vi "Main Voice.vi"() -> ()   [LabVIEW 2018]
uses:
  <vilib>/LabVIEW Hacker/LINX/Private/Type Defs/User Platform.ctl
  <vilib>/LabVIEW Hacker/LINX/Private/Type Defs/Interface.ctl
  <vilib>/LabVIEW Hacker/LINX/Public/Peripherals/Digital/Digital Write 1 Chan.vi
  <vilib>/LabVIEW Hacker/LINX/Public/Peripherals/Digital/Digital Write N Chans.vi
  <vilib>/LabVIEW Hacker/LINX/Private/Local IO/LinxDigitalWrite.vi
  <vilib>/LabVIEW Hacker/LINX/Public/Utilities/Check Channel.vi
  <vilib>/LabVIEW Hacker/LINX/Private/Utilties/Generate Error.vi
  <vilib>/LabVIEW Hacker/LINX/LMH-LINX.lvlib
panel:
  out "Command":string[](array[string])
  in  "Error In":errorcluster
  out "Error Out":errorcluster
  in  "Exit":bool
  out "Voice Command":string
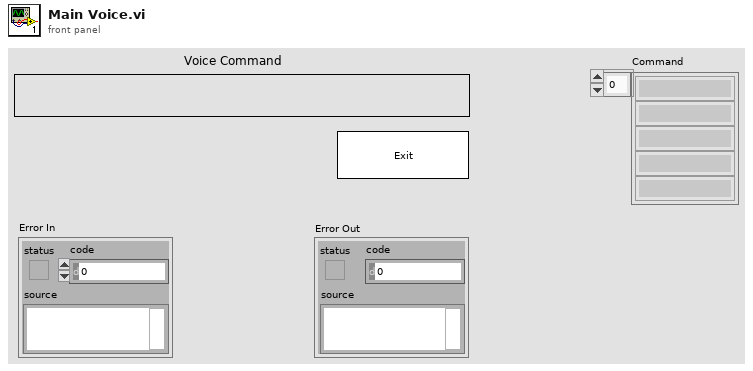
[diagram p1: front panel]
types:
  T1 = typedef "LMH-LINX.lvlib/Interface.ctl" = enum16{"Serial", "TCP"}
  T2 = typedef "LMH-LINX.lvlib/User Platform.ctl" = enum16{"Default", "Remote", "Local"}
  T3 = typedef "LMH-LINX.lvlib/LINX Ref.ctl" = cluster{"IO":T4, "Interface":T1, "LINX Device Config":T5}
  T4 = typedef "LMH-LINX.lvlib/Platform.ctl" = enum16{"Remote", "Local"}
  T5 = typedef "LMH-LINX.lvlib/Device.lvlib/LINX Device Config.ctl" = cluster{"Interface":T1, "COM Port":refnum<visa-resource-name>, "TCP Configuration":T6, "Device Family":u8, "Device ID":u8, "Device Name":string, "TCP Ref":refnum<k5>, "Channels":T7}
  T6 = typedef "LMH-LINX.lvlib/Device.lvlib/TCP Config.ctl" = cluster{"IP Address":string, "Port":u16}
  T7 = typedef "LMH-LINX.lvlib/Channels.ctl" = cluster{"DI":u8[], "DO":u8[], "AI":u8[], "AO":u8[], "PWM":u8[], "QE":u8[], "UART":u8[], "I2C 2":u8[], "SPI":u8[], "CAN":u8[], "Servo":u8[], "AI Ref (V)":dbl, "AI Resolution (Bits)":u8, "AO Ref (V)":dbl, "AO Resolution (Bits)":u8}
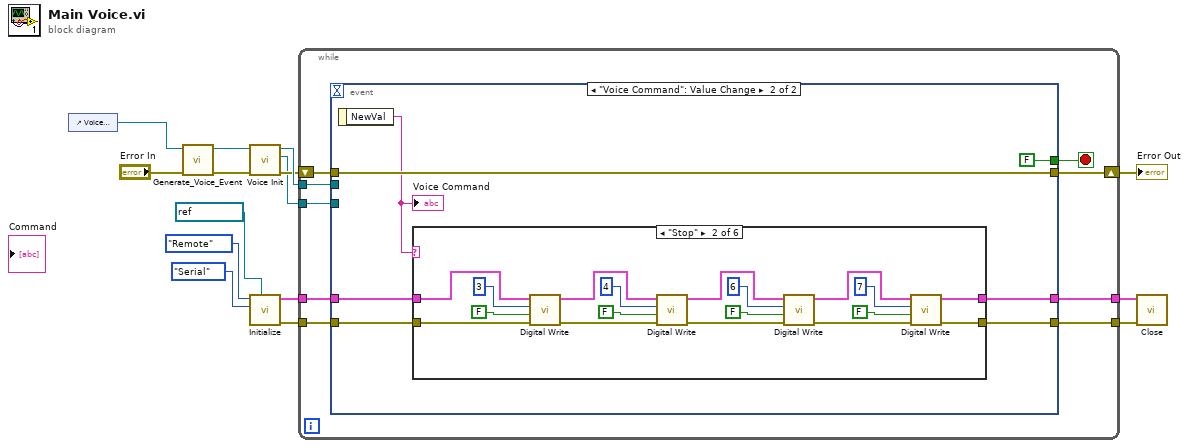
[diagram p0: block diagram]
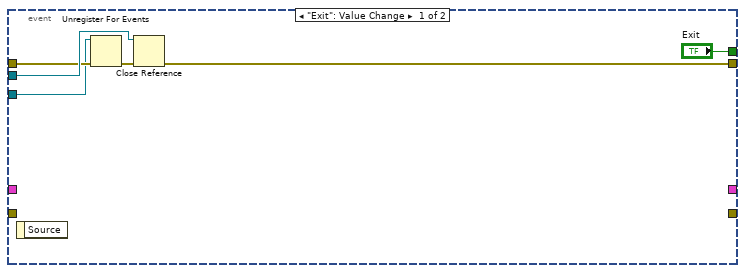
[diagram p2: hidden frame]
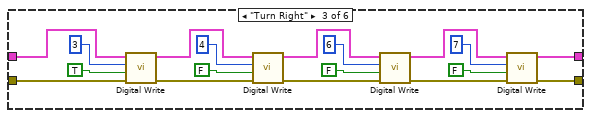
[diagram p4: hidden frame]
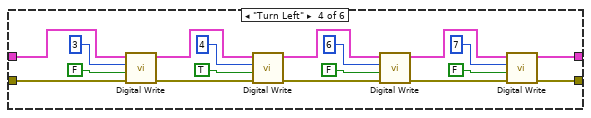
[diagram p5: hidden frame]
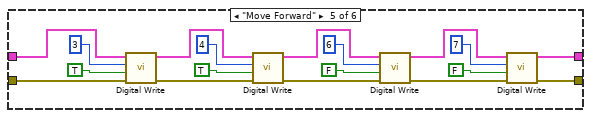
[diagram p6: hidden frame]
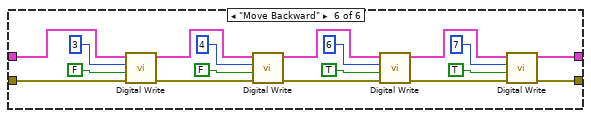
[diagram p7: hidden frame]
diagram:
  n1 = control-ref of="Voice Command"() -> (w14:refnum<vi>)
  n2 = call "Generate_Voice_Event.vi"("Error In"="Error In", "String in"=w14) -> ("Error Out"=w13:errorcluster, "String out"=w15:refnum<vi>)  [unwired: 8 in]
  n3 = call "Voice Init.vi"("Error In"=w13, "Text"=w15) -> ("Error Out"=w11:errorcluster, "Event Callback"=w8:refnum<k27>, "Reference"=w12:refnum<k24>)  [unwired: 7 in]
  n4 = call <vilib>:"Initialize.vi"("Serial Port"=refnum<visa-resource-name> "COM19", "Interface"=Interface."Serial", "IO"=User_Platform."Remote" ("Platform")) -> ("Error Out"=w6:errorcluster, "LINX Resource"=w7:T3)  [unwired: 6 in, 1 out]
  n5 = while {
    tunnel: w12 -> [w23]
    shift-right: [w21] -> w10
    shift-left: w11 -> [w22]
    tunnel: w8 -> [w20]
    tunnel: w7 -> [w19]
    tunnel: w6 -> [w18]
    tunnel: [w17] -> w5
    tunnel: [w16] -> w4
    stop <- w24 stop-if-true
    n6 = event shown="[1] \"Voice Command\": Value Change" {
      selector: _ -> [_ _]
      dyn-events: _ -> [_ _]
      timeout: _ -> [_ _]
      tunnel: ["Exit" FALSE ("Exit")] -> w24
      tunnel: w23 -> [w29 _]
      tunnel: w22 -> [w27 w37]
      tunnel: [w26 w37] -> w21
      tunnel: w20 -> [w25 _]
      tunnel: w19 -> [_ w34]
      tunnel: w18 -> [_ w33]
      tunnel: [_ w32] -> w17
      tunnel: [_ w31] -> w16
      event "Exit": Value Change {
        n7 = event-data() -> ()  [unwired: 1 in, 1 out]
        n8 = Unregister For Events(event registration refnum=w25, error in=w27) -> (error out=w28:errorcluster)
        n9 = Close Reference(reference=w29, error in (no error)=w28) -> (error out=w26:errorcluster)
      }
      event "Voice Command": Value Change {
        n10 = event-data() -> ("NewVal"=w35:string)  [unwired: 1 in]
        "Voice Command" <- w35
        n11 = case shown="\"Stop\"" w35 {
          tunnel: w34 -> [w39 w46 w64 w82 w100 w118]
          tunnel: w33 -> [w38 w45 w63 w81 w99 w117]
          tunnel: [w39 w41 w62 w77 w95 w113] -> w32
          tunnel: [w38 w40 w61 w76 w94 w112] -> w31
          frame Default {
          }
          frame "Stop" {
            n12 = call-poly <vilib>:"Digital Write.vi"("Error In"=w45, "Output Value"=FALSE, "DO Channel"=u8 3, "LINX Resource"=w46) -> ("Error Out"=w44:errorcluster, "LINX Resource"=w47:T3)  [unwired: 6 in]
            n13 = call-poly <vilib>:"Digital Write.vi"("Error In"=w44, "Output Value"=FALSE, "DO Channel"=u8 4, "LINX Resource"=w47) -> ("Error Out"=w43:errorcluster, "LINX Resource"=w48:T3)  [unwired: 6 in]
            n14 = call-poly <vilib>:"Digital Write.vi"("Error In"=w43, "Output Value"=FALSE, "DO Channel"=u8 6, "LINX Resource"=w48) -> ("Error Out"=w42:errorcluster, "LINX Resource"=w49:T3)  [unwired: 6 in]
            n15 = call-poly <vilib>:"Digital Write.vi"("Error In"=w42, "Output Value"=FALSE, "DO Channel"=u8 7, "LINX Resource"=w49) -> ("Error Out"=w40:errorcluster, "LINX Resource"=w41:T3)  [unwired: 6 in]
          }
          frame "Turn Right" {
            n16 = call-poly <vilib>:"Digital Write.vi"("Error In"=w63, "Output Value"=TRUE, "DO Channel"=u8 3, "LINX Resource"=w64) -> ("Error Out"=w60:errorcluster, "LINX Resource"=w75:T3)  [unwired: 6 in]
            n17 = call-poly <vilib>:"Digital Write.vi"("Error In"=w60, "Output Value"=FALSE, "DO Channel"=u8 4, "LINX Resource"=w75) -> ("Error Out"=w59:errorcluster, "LINX Resource"=w74:T3)  [unwired: 6 in]
            n18 = call-poly <vilib>:"Digital Write.vi"("Error In"=w59, "Output Value"=FALSE, "DO Channel"=u8 6, "LINX Resource"=w74) -> ("Error Out"=w58:errorcluster, "LINX Resource"=w73:T3)  [unwired: 6 in]
            n19 = call-poly <vilib>:"Digital Write.vi"("Error In"=w58, "Output Value"=FALSE, "DO Channel"=u8 7, "LINX Resource"=w73) -> ("Error Out"=w61:errorcluster, "LINX Resource"=w62:T3)  [unwired: 6 in]
          }
          frame "Turn Left" {
            n20 = call-poly <vilib>:"Digital Write.vi"("Error In"=w81, "Output Value"=FALSE, "DO Channel"=u8 3, "LINX Resource"=w82) -> ("Error Out"=w80:errorcluster, "LINX Resource"=w83:T3)  [unwired: 6 in]
            n21 = call-poly <vilib>:"Digital Write.vi"("Error In"=w80, "Output Value"=TRUE, "DO Channel"=u8 4, "LINX Resource"=w83) -> ("Error Out"=w79:errorcluster, "LINX Resource"=w84:T3)  [unwired: 6 in]
            n22 = call-poly <vilib>:"Digital Write.vi"("Error In"=w79, "Output Value"=FALSE, "DO Channel"=u8 6, "LINX Resource"=w84) -> ("Error Out"=w78:errorcluster, "LINX Resource"=w85:T3)  [unwired: 6 in]
            n23 = call-poly <vilib>:"Digital Write.vi"("Error In"=w78, "Output Value"=FALSE, "DO Channel"=u8 7, "LINX Resource"=w85) -> ("Error Out"=w76:errorcluster, "LINX Resource"=w77:T3)  [unwired: 6 in]
          }
          frame "Move Forward" {
            n24 = call-poly <vilib>:"Digital Write.vi"("Error In"=w99, "Output Value"=TRUE, "DO Channel"=u8 3, "LINX Resource"=w100) -> ("Error Out"=w98:errorcluster, "LINX Resource"=w101:T3)  [unwired: 6 in]
            n25 = call-poly <vilib>:"Digital Write.vi"("Error In"=w98, "Output Value"=TRUE, "DO Channel"=u8 4, "LINX Resource"=w101) -> ("Error Out"=w97:errorcluster, "LINX Resource"=w102:T3)  [unwired: 6 in]
            n26 = call-poly <vilib>:"Digital Write.vi"("Error In"=w97, "Output Value"=FALSE, "DO Channel"=u8 6, "LINX Resource"=w102) -> ("Error Out"=w96:errorcluster, "LINX Resource"=w103:T3)  [unwired: 6 in]
            n27 = call-poly <vilib>:"Digital Write.vi"("Error In"=w96, "Output Value"=FALSE, "DO Channel"=u8 7, "LINX Resource"=w103) -> ("Error Out"=w94:errorcluster, "LINX Resource"=w95:T3)  [unwired: 6 in]
          }
          frame "Move Backward" {
            n28 = call-poly <vilib>:"Digital Write.vi"("Error In"=w117, "Output Value"=FALSE, "DO Channel"=u8 3, "LINX Resource"=w118) -> ("Error Out"=w116:errorcluster, "LINX Resource"=w119:T3)  [unwired: 6 in]
            n29 = call-poly <vilib>:"Digital Write.vi"("Error In"=w116, "Output Value"=FALSE, "DO Channel"=u8 4, "LINX Resource"=w119) -> ("Error Out"=w115:errorcluster, "LINX Resource"=w120:T3)  [unwired: 6 in]
            n30 = call-poly <vilib>:"Digital Write.vi"("Error In"=w115, "Output Value"=TRUE, "DO Channel"=u8 6, "LINX Resource"=w120) -> ("Error Out"=w114:errorcluster, "LINX Resource"=w121:T3)  [unwired: 6 in]
            n31 = call-poly <vilib>:"Digital Write.vi"("Error In"=w114, "Output Value"=TRUE, "DO Channel"=u8 7, "LINX Resource"=w121) -> ("Error Out"=w112:errorcluster, "LINX Resource"=w113:T3)  [unwired: 6 in]
          }
        }
      }
    }
  }
  "Error Out" <- w10
  n32 = call <vilib>:"Close.vi"("Error In"=w4, "LINX Resource"=w5) -> ()  [unwired: 9 in, 1 out]
